vi "Microscopy.Detect Trigger Edge.vi"(7 "Trigger Configuration":T3={"Acq Trigger Type"=enum."Software", "Acq Trigger On Falling Edge"=FALSE, "Acq Software Trigger from Host"=FALSE, "Period Clock Type"=enum."Software", "Period Clock On Falling Edge"=FALSE, "Period Software Trigger from Host"=FALSE, "Advance Trigger Type"=enum."Software", "Advance Trigger On Falling Edge"=FALSE, "Advance Software Trigger from Host"=FALSE, "Stop Trigger Type"=enum."Software", "Stop Trigger On Falling Edge"=FALSE, "Stop Software Trigger from Host"=FALSE}, 8 "Data Valid In":bool, 10 "Trigger Signals":T1, 11 "Analog Channel Data":T4=[0, 0, 0, 0]) -> (0 "Data Valid Out":bool, 1 "Trigger Edges":T1, 3 "Analog Channel Data":T4)   [LabVIEW 2014]
doc: "This VI detects rising edge on a select trigger Type.\n\nThe trigger type is selected from the Host. The trigger types can be\n1) External Digital Trigger\n2) Software Trigger from Host\n3) Immediate Trigger"
uses:
  Adapter Module Specific/Multi-Channel Analog Input Data.ctl
  Adapter Module Specific/Trigger Signals.ctl
  Adapter Module Specific/Trigger Type.ctl
panel:
  # "Copyright 2014 Vidrio Technologies\nScanImage 5 software is licensed under the Apache License, Version 2.0 (the \"License\"); you may not use any files contained\nwithin the ScanImage 5 release except in compliance with the License. You may obtain a copy of the License at\n http://www.apache.org/licenses/LICENSE-2.0\nUnless required by applicable law or agreed to in writing, software distributed under the License is distributed on an\n\"AS IS\" BASIS, WITHOUT WARRANTIES OR CONDITIONS OF ANY KIND, either express or implied. See the License for the\n specific language governing permissions and limitations under the License."
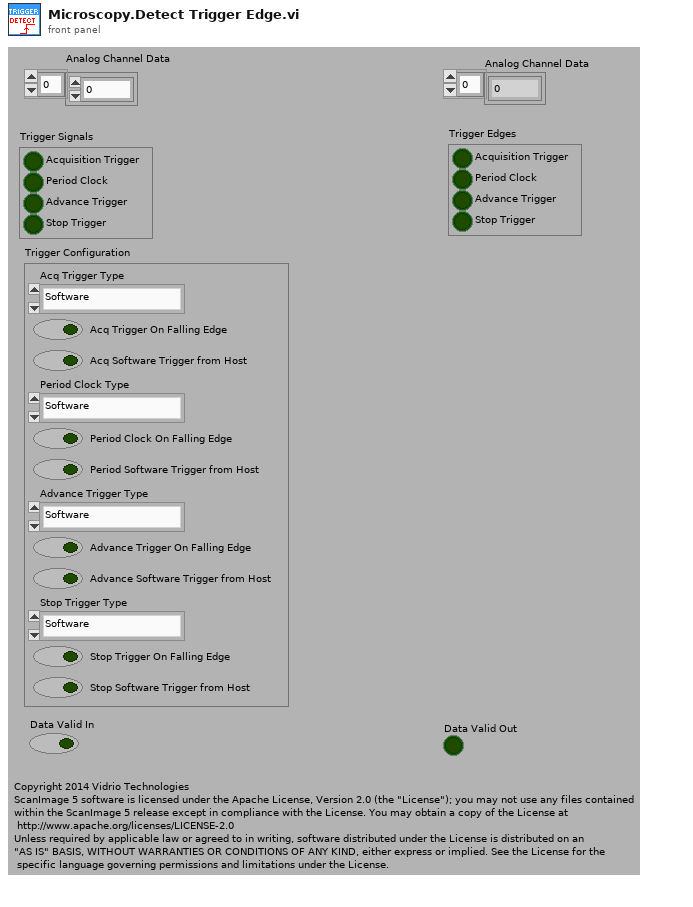
[diagram p1: front panel]
types:
  T1 = typedef "Trigger Signals.ctl" = cluster{"Acquisition Trigger":bool, "Period Clock":bool, "Advance Trigger":bool, "Stop Trigger":bool}
  T2 = typedef "Trigger Type.ctl" = enum8{"External", "Software", "Immediate", "External or Software", "None"}
  T3 = cluster{"Acq Trigger Type":T2, "Acq Trigger On Falling Edge":bool, "Acq Software Trigger from Host":bool, "Period Clock Type":T2, "Period Clock On Falling Edge":bool, "Period Software Trigger from Host":bool, "Advance Trigger Type":T2, "Advance Trigger On Falling Edge":bool, "Advance Software Trigger from Host":bool, "Stop Trigger Type":T2, "Stop Trigger On Falling Edge":bool, "Stop Software Trigger from Host":bool}
  T4 = typedef "Multi-Channel Analog Input Data.ctl" = i16[]
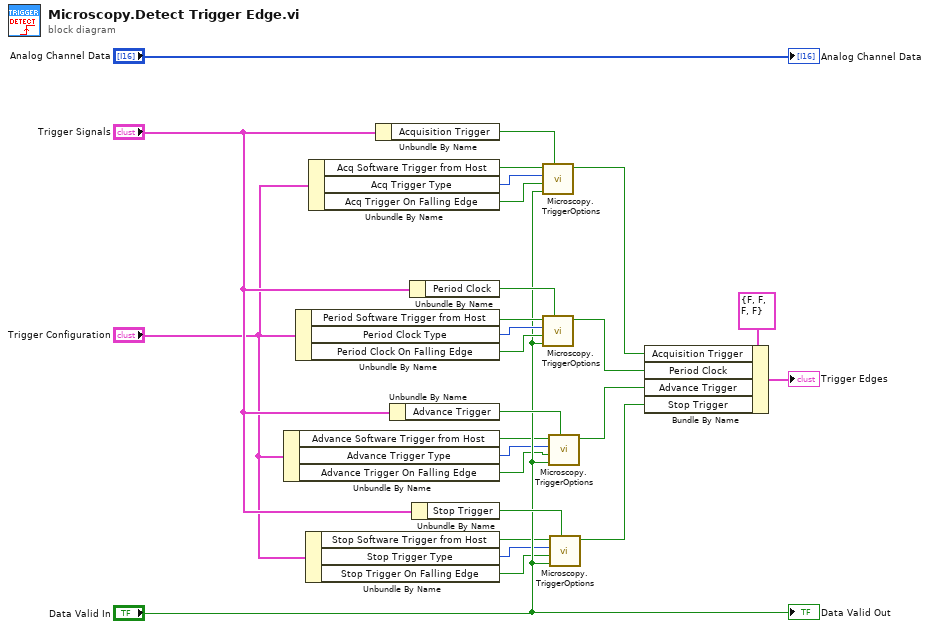
[diagram p0: block diagram]
diagram:
  n1 = Unbundle By Name("Trigger Configuration") -> ("Advance Software Trigger from Host"=w3:bool, "Advance Trigger Type"=w2:T2, "Advance Trigger On Falling Edge"=w1:bool)
  n2 = Unbundle By Name("Trigger Configuration") -> ("Period Software Trigger from Host"=w17:bool, "Period Clock Type"=w16:T2, "Period Clock On Falling Edge"=w15:bool)
  n3 = Unbundle By Name("Trigger Configuration") -> ("Stop Software Trigger from Host"=w6:bool, "Stop Trigger Type"=w5:T2, "Stop Trigger On Falling Edge"=w4:bool)
  n4 = Unbundle By Name("Trigger Configuration") -> ("Acq Software Trigger from Host"=w20:bool, "Acq Trigger Type"=w19:T2, "Acq Trigger On Falling Edge"=w18:bool)
  n5 = Unbundle By Name("Trigger Signals") -> ("Acquisition Trigger"=w21:bool)
  n6 = Unbundle By Name("Trigger Signals") -> ("Advance Trigger"=w13:bool)
  n7 = Unbundle By Name("Trigger Signals") -> ("Period Clock"=w14:bool)
  n8 = Unbundle By Name("Trigger Signals") -> ("Stop Trigger"=w12:bool)
  n9 = call "Microscopy.TriggerOptions.vi"("Trigger In"=w21, "Data Valid in"="Data Valid In", "Trigger Falling Edge Detect"=w18, "Trigger Type"=w19, "Software Trigger from Host"=w20) -> ("trigger edge"=w23:bool)  [unwired: 5 in, 1 out]
  n10 = call "Microscopy.TriggerOptions.vi"("Trigger In"=w14, "Data Valid in"="Data Valid In", "Trigger Falling Edge Detect"=w15, "Trigger Type"=w16, "Software Trigger from Host"=w17) -> ("trigger edge"=w22:bool)  [unwired: 5 in, 1 out]
  n11 = call "Microscopy.TriggerOptions.vi"("Trigger In"=w13, "Data Valid in"="Data Valid In", "Trigger Falling Edge Detect"=w1, "Trigger Type"=w2, "Software Trigger from Host"=w3) -> ("trigger edge"=w8:bool)  [unwired: 5 in, 1 out]
  n12 = call "Microscopy.TriggerOptions.vi"("Trigger In"=w12, "Data Valid in"="Data Valid In", "Trigger Falling Edge Detect"=w4, "Trigger Type"=w5, "Software Trigger from Host"=w6) -> ("trigger edge"=w7:bool)  [unwired: 5 in, 1 out]
  n13 = Bundle By Name(cluster=T1 {"Acquisition Trigger"=FALSE, "Period Clock"=FALSE, "Advance Trigger"=FALSE, "Stop Trigger"=FALSE} ("Trigger Edge"), "Acquisition Trigger"=w23, "Period Clock"=w22, "Advance Trigger"=w8, "Stop Trigger"=w7) -> (→"Trigger Edges":T1)
  "Data Valid Out" <- "Data Valid In"
  "Analog Channel Data" <- "Analog Channel Data"
